vi "art联动采集V4.8.2.vi"() -> ()   [LabVIEW 2016]
uses:
  <vilib>/Instr/_visa.llb/VISA Configure Serial Port (Instr).vi
  <vilib>/Utility/file.llb/Write Delimited Spreadsheet (DBL).vi
panel:
  out "水平进度条":u8(slide) scale=0.0..100.0
  out "x+y 3":dbl=3.0
  in  "分层图查看":bool
  in  "hDevice 2":i32
  in  "逐行扫描":bool
  in  "定位模式":bool
  in  "X终点":dbl
  in  "Y终点":dbl
  in  "高级设置":bool
  in  "Y轴回零速度":dbl=15000.0
  in  "X轴回零速度":dbl=15000.0
  in  "细分设置":dbl=8.0
  in  "等待时间":u32=40
  in  "文件保存":path=path "C:/Users/H301/Desktop/art采集实验数据" caption="保存路径"
  out "已用时（s）":dbl format="%<%H:%M:%S>t"
  out "error out":errorcluster caption="错误输出"
  in  "退出扫描(Esc)":bool
  in  "N_Length":i32=16384
  out "M_Length":i32
  out "hDevice":i32=241832032
  out "pulDDR2Length":u32=256
  out "毫秒计时值":u32=3586537
  out "数组":dbl[][](array[numeric])=[[58819.77200735986, 88200.32943600747]]
  out "强度图":dbl[][](graph)=[[58819.77200735986, 88200.32943600747]]
  out "judge":dbl
  out "Xloop":dbl
  out "幅频谱":dbl[](graph)
  out "时域谱":dbl[](graph)
  out "错误输出":errorcluster
  in  "启动":bool
  in  "逐点扫描":bool
  in  "X归零":bool
  in  "Y归零":bool
  in  "Y起点":dbl
  in  "Y轴速度":dbl=9000.0
  in  "X轴速度":dbl=9000.0
  out "电机状态":bool
  in  "电机端口":refnum<visa-resource-name>="COM6"
  out "Yloop":dbl=1.0
  out "X扫描范围":dbl=150.0
  out "Y扫描范围":dbl=75.0
  out "Y序":i32
  in  "X起点":dbl
  out "Y(mm)":dbl
  out "x+y 2":dbl=3.0
  in  "Y:":dbl=1.0
  in  "精度":dbl=0.001
  in  "电机急停":bool
  out "X（mm）":dbl
  out "x+y":dbl=1.0
  in  "X:":dbl=1.0
  # "实时坐标"
  # "时域谱"
  # "频域谱"
  # "归零"
  # "扫描区域"
  # "扫描步进(mm)"
  # "X:"
  # "~"
  # "Y:"
  # "~"
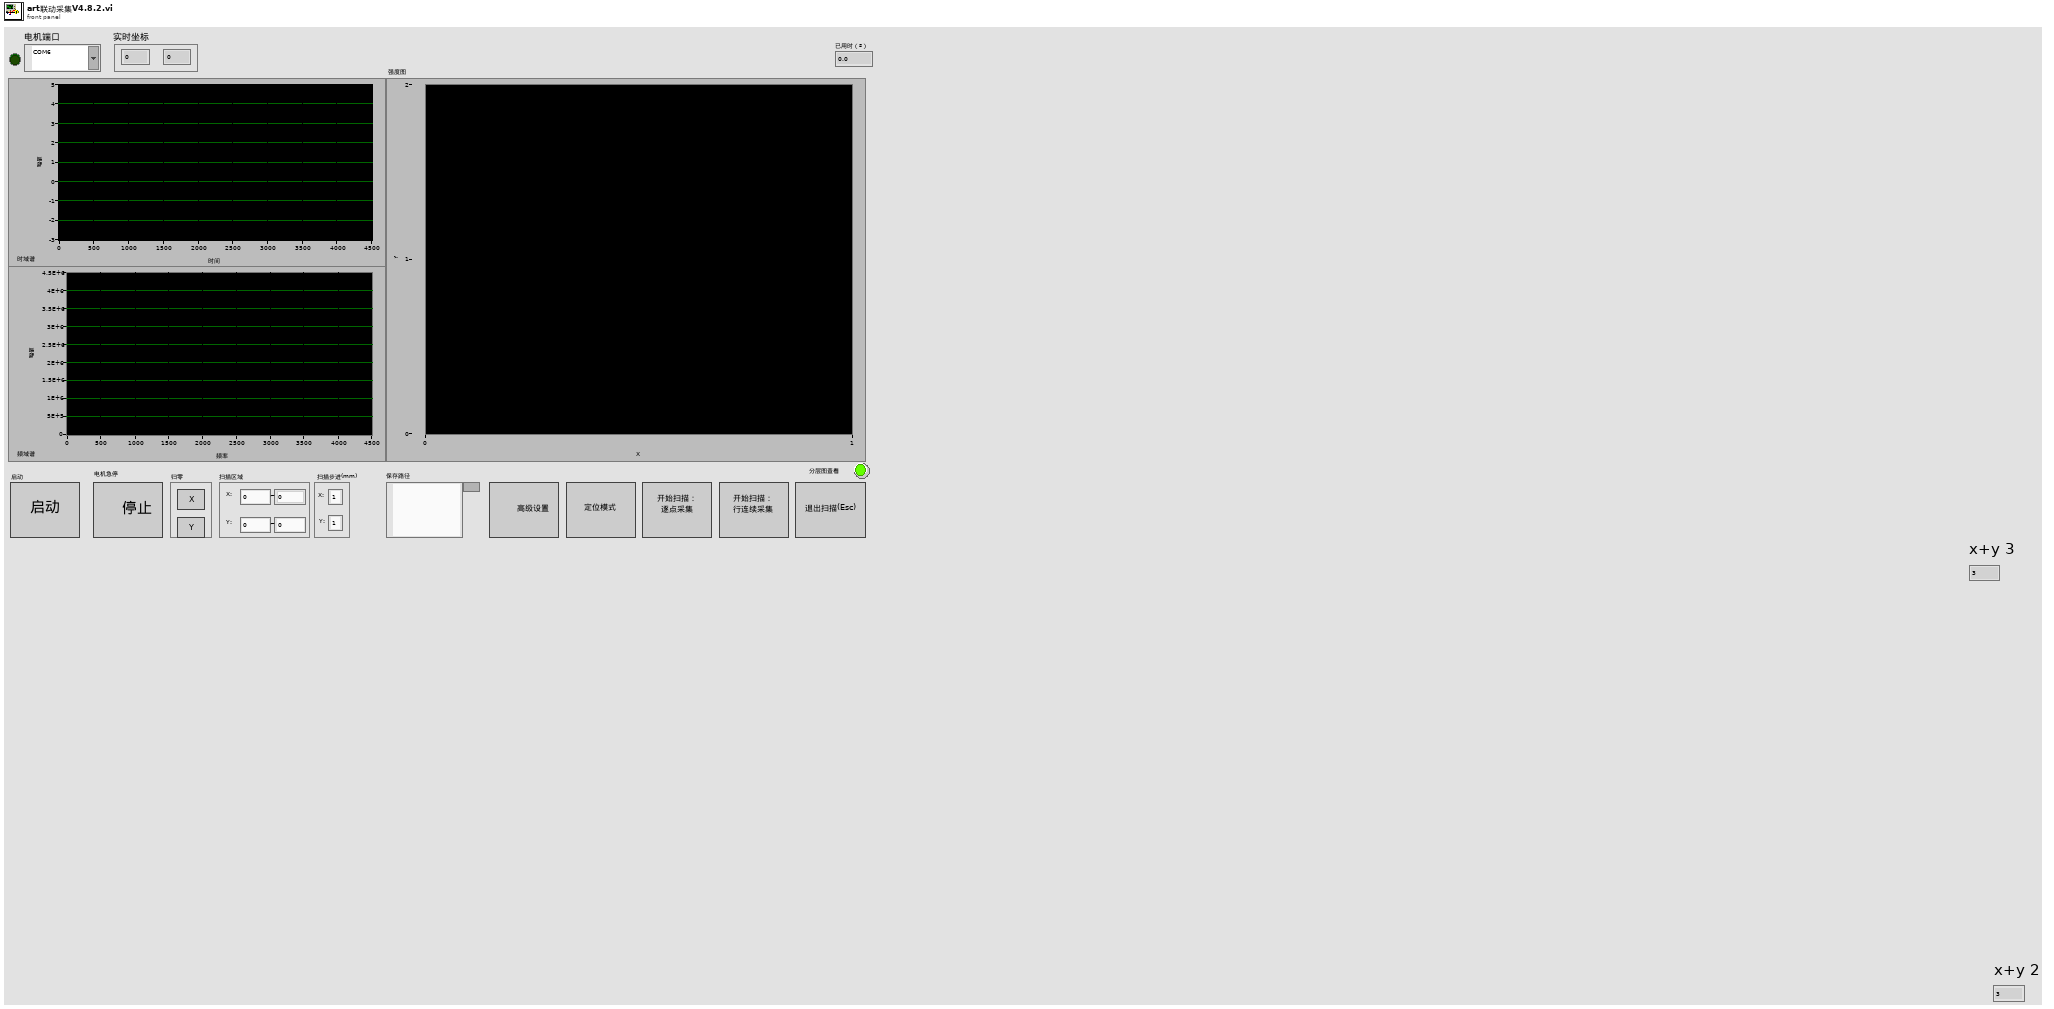
[diagram p1: front panel]
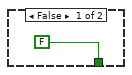
[diagram p2: hidden frame]
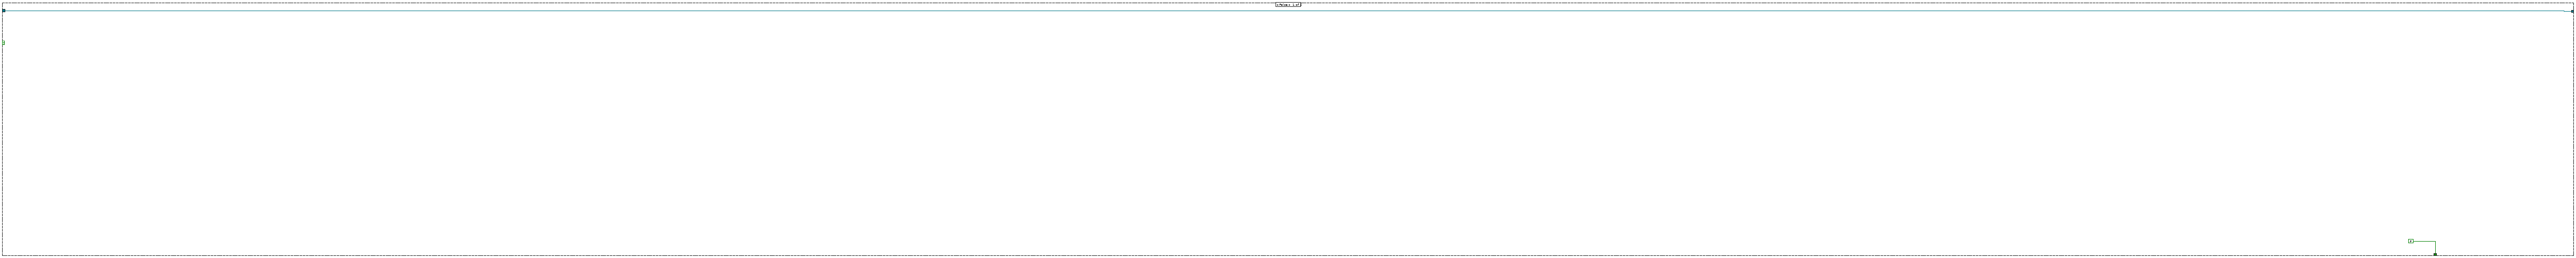
[diagram p3: hidden frame]
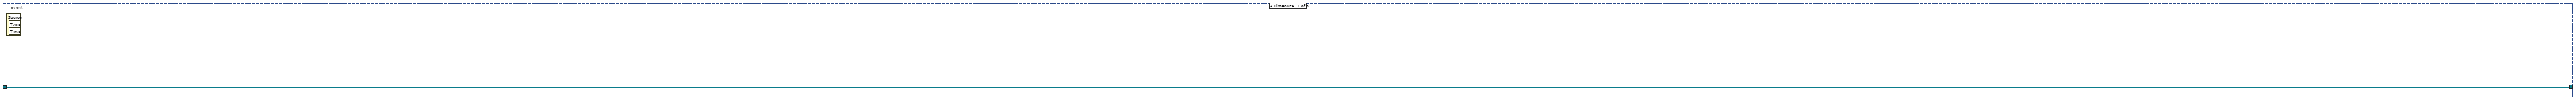
[diagram p4: hidden frame]
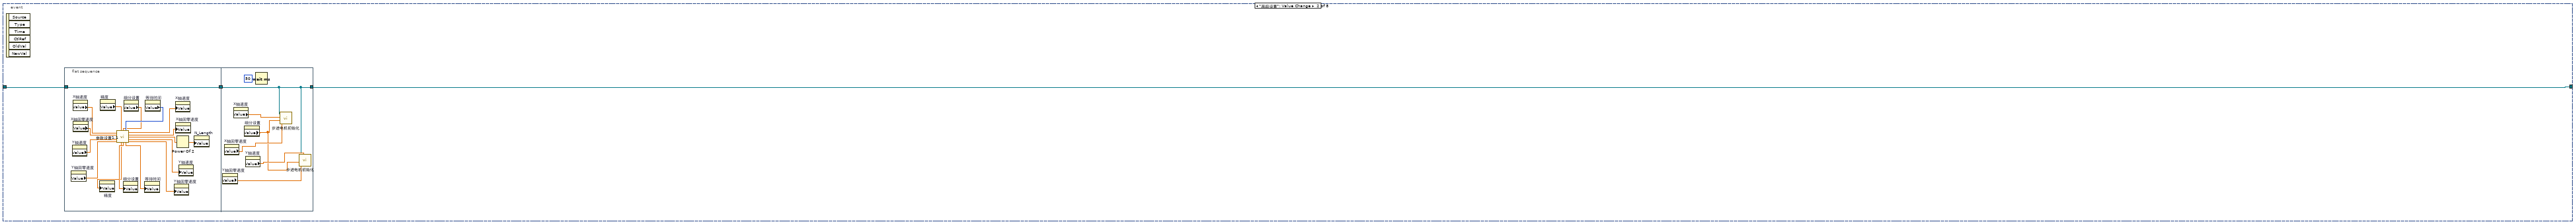
[diagram p5: hidden frame]
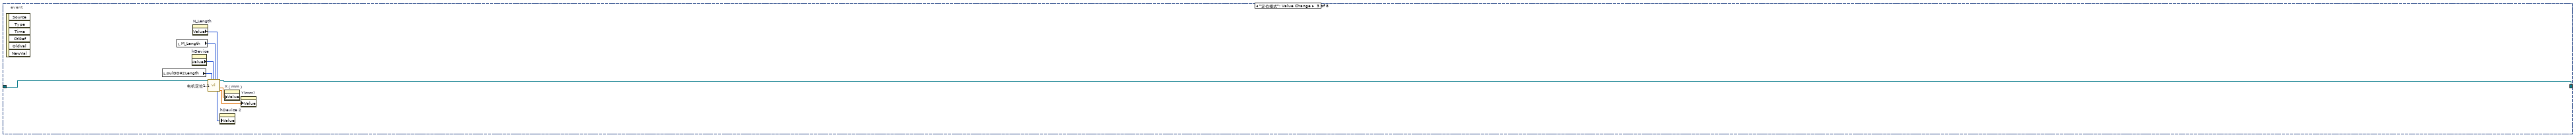
[diagram p6: hidden frame]
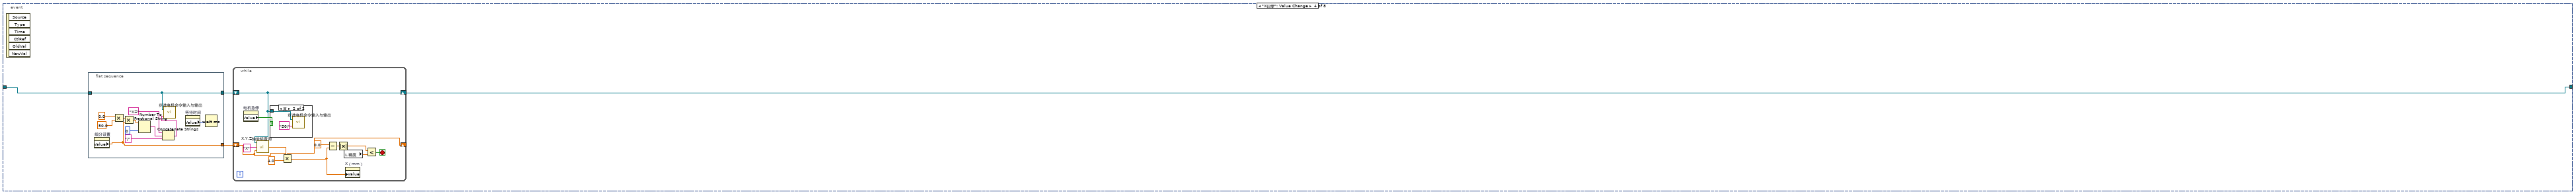
[diagram p7: hidden frame]
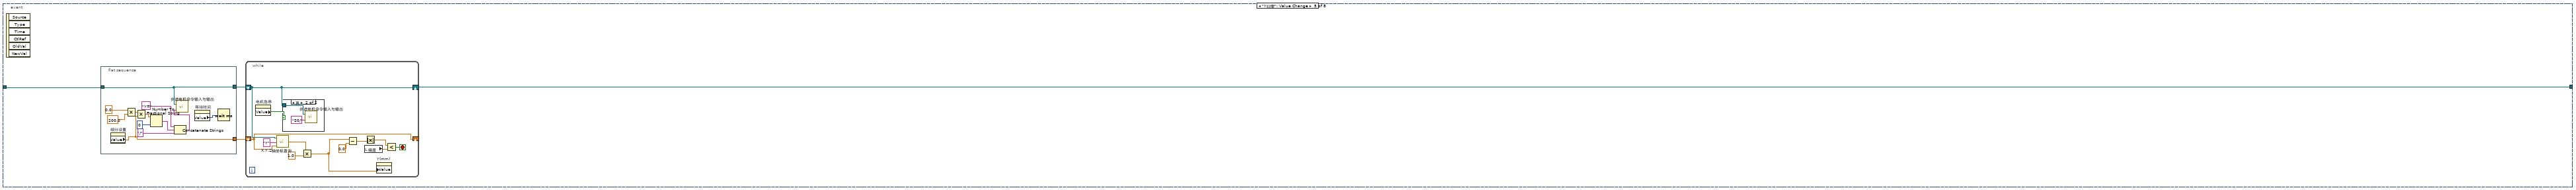
[diagram p9: hidden frame]
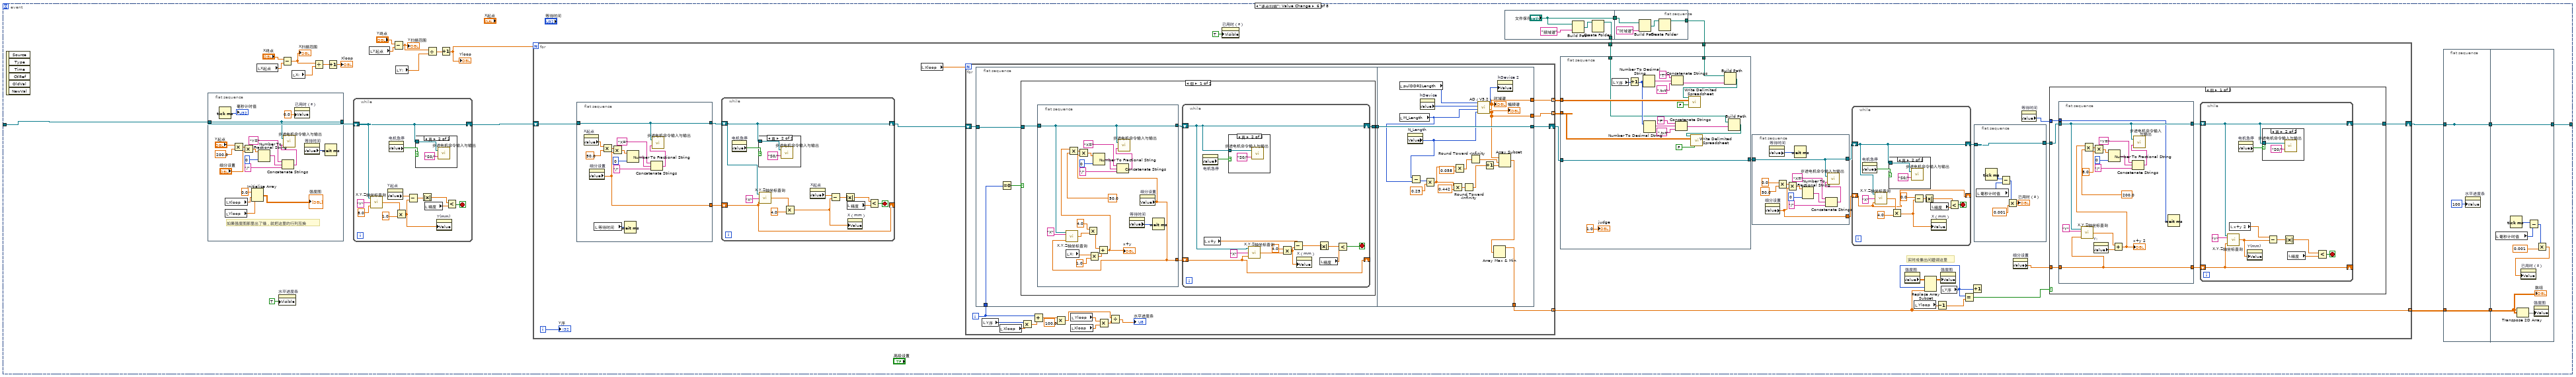
[diagram p11: hidden frame]
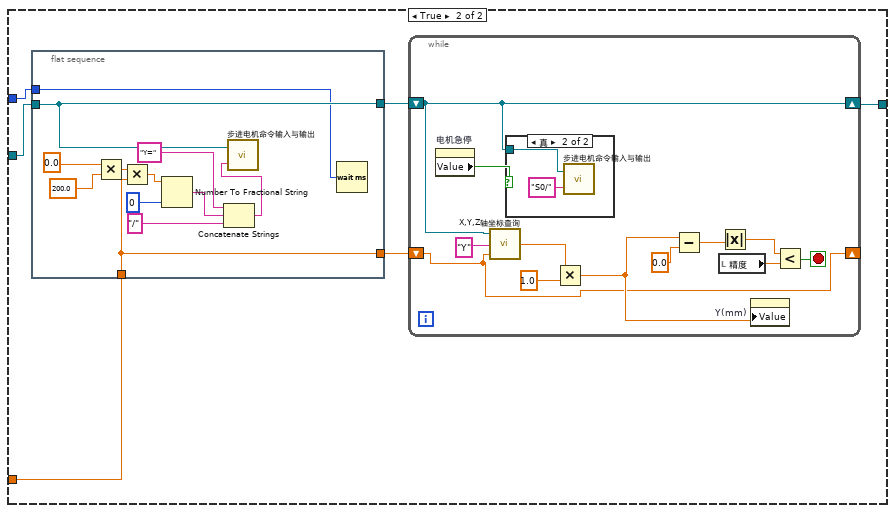
[diagram p16: hidden frame]
diagram:
  n1 = for {
    N: 255 -> [_]
    tunnel: [w12] -> w9 mode=indexing
    i -> [w12]
  }
  n2 = To Unsigned Byte Integer(number=w9) -> (unsigned 8bit integer=w6:u8[])
  n3 = Join Numbers(hi=u16 0, lo=w6) -> ((hi.lo)=w8:u32[])
  n4 = Join Numbers(hi=w6, lo=w6) -> ((hi.lo)=w5:u16[])
  n5 = Join Numbers(hi=w8, lo=w5) -> ((hi.lo)=w4:u64[])
  n6 = property on="强度图" class="IntGraph (严格)"("Color Table"=w4) -> ()  [unwired: 2 in, 2 out]
  n7 = property on="水平进度条" class="Slide (严格)"("Visible"=FALSE ("可见")) -> ()  [unwired: 2 in, 2 out]
  n8 = while {
    stop <- w13 stop-if-true
    n9 = case shown="真" "启动" {
      tunnel: [FALSE ("ESC") w21] -> w13
      frame False {
      }
      frame True {
        w32 = 0  # OutClockSource
        w33 = 0  # bClockSourceDir
        w35 = 10000000  # Frequency
        w36 = 0  # ClockSource
        w37 = 0  # TrigLevelVolt
        w25 = 1
        w38 = 0  # TriggerDir
        w39 = 0  # TriggerSource
        w40 = 0  # ATRTriggerChannel
        w41 = 0  # TriggerMode
        w26 = 0  # M_Length
        w42 = 1  # CouplingType
        w43 = 0  # DeviceLgcID
        w53 = u16 0 items=["无", "XON/XOFF", "RTS/CTS", "XON/XOFF & RTS/CTS", "DTR/DSR", "XON/XOFF & DTR/DSR"] ("flow control (0:none)")
        w54 = u16 10 items=["1.0"=10, "1.5"=15, "2.0"=20] ("stop bits (10: 1 bit)")
        # "3"
        # "2"
        # "1"
        n10 = call-poly "VISA Configure Serial Port"("VISA resource name"="电机端口", "baud rate (9600)"=u32 9600, "data bits (8)"=u16 8, "parity (0:none)"=enum16{"None", "Odd", "Even", "Mark", "Space"}."None", "stop bits (10: 1 bit)"=w54, "flow control (0:none)"=w53) -> ("VISA resource name out"=w45:refnum<visa-resource-name>, "error out"=→"error out":errorcluster)  [unwired: 1 in, 7 out]
        n11 = Build Array "InputRange"(w25, w25, w25, w25) -> (w24:i32[])
        n12 = dll-call lib="PTH2aabs CUsersH301Desktopart闭环扫描程序采集卡控制INFamd64PCI8502_32.dll" fn="PCI8502_CreateDevice" label="CreateDevice"("DeviceLgcID"=w43) -> (w30:i32)  [unwired: 4 in, 2 out]
        n13 = property on="细分设置" class="DigNum (严格)"() -> ("Value"=w20:dbl)  [unwired: 2 in, 2 out]
        n14 = Build Array (concatenate) "InitDeviceAD"(w35, w24, w42, w26, "N_Length", w41, w40, w39, w38, w37, w36, w33, w32) -> (w34:i32[])
        n15 = call "步进电机初始化.vi"("回零速度"="X轴回零速度", "细分设置"=w20, "X轴速度"="X轴速度", "串口通信端口"=w45) -> ()  [unwired: 2 in, 1 out]
        n16 = dll-call lib="PTH2aabs CUsersH301Desktopart闭环扫描程序采集卡控制INFamd64PCI8502_32.dll" fn="PCI8502_GetDDR2Length" label="GetDDR2Length"("hDevice"=w30, "pulDDR2Length"=u32 0) -> ("hDevice"=w29:i32, "pulDDR2Length"=→"pulDDR2Length":u32)  [unwired: 4 in, 2 out]
        n17 = call "步进电机初始化.vi"("Y轴速度"="Y轴速度", "回零速度"="Y轴回零速度", "细分设置"=w20, "串口通信端口"=w45) -> ()  [unwired: 2 in, 1 out]
        n18 = call "步进电机命令输入与输出.vi"("输入字符串"="?R/", "串口通信端口"=w45) -> ("返回字符串"=w50:string)
        n19 = dll-call lib="PTH2aabs CUsersH301Desktopart闭环扫描程序采集卡控制INFamd64PCI8502_32.dll" fn="PCI8502_InitDeviceAD" label="InitDeviceAD"("hDevice"=w29, "pADPara"=w34) -> ("hDevice"=→"hDevice":i32)  [unwired: 5 in, 2 out]
        n20 = String Subset(string=w50, offset (0)=0 ("偏移量(0)"), length (rest)=2 ("长度（剩余）")) -> (substring=w47:string)
        n21 = Equal?(x=w47, y="OK") -> (x = y?=w44:bool)
        "电机状态" <- w44
        n22 = case shown="真" w44 {
          tunnel: w45 -> [w65 w68]
          tunnel: [w65 w66] -> w22
          tunnel: [FALSE ("ESC") w67] -> w21
          frame False {
          }
          frame True {
            n23 = while {
              tunnel: ["退出扫描(Esc)"] -> w67
              shift-right: [w71] -> w66
              shift-left: w68 -> [w76]
              stop <- "退出扫描(Esc)" stop-if-true
              n24 = property on="水平进度条" class="Slide (严格)"("Visible"=FALSE ("可见")) -> ()  [unwired: 2 in, 2 out]
              n25 = property on="高级设置" class="Bool"("Visible"=TRUE ("可见")) -> ()  [unwired: 2 in, 2 out]
              n26 = property on="定位模式" class="Bool"("Visible"=TRUE ("可见")) -> ()  [unwired: 2 in, 2 out]
              n27 = property on="水平进度条" class="Slide (严格)"("Value"=u8 0 ("水平进度条")) -> ()  [unwired: 2 in, 2 out]
              n28 = event shown="[6] \"逐行扫描\": 值改变" {
                selector: _ -> [_ _ _ _ _ _ _ _]
                dyn-events: _ -> [_ _ _ _ _ _ _ _]
                timeout: 1 -> [_ _ _ _ _ _ _ _]
                tunnel: w76 -> [w77 w80 w113 w117 w147 w198 w507 w735]
                tunnel: [w77 w79 w112 w115 w145 w193 w510 w734] -> w71
                event Timeout {
                  n29 = event-data() -> ()  [unwired: 1 in, 3 out]
                }
                event "高级设置": Value Change {
                  n30 = event-data() -> ()  [unwired: 1 in, 6 out]
                  n31 = flat-sequence {
                    tunnel: w80 -> [w83]
                    tunnel: [w83] -> w78
                    tunnel: [w99] -> w79
                    tunnel: w78 -> [w99]
                    frame #0 {
                      n32 = property on="Y轴回零速度" class="DigNum (严格)"() -> ("Value"=w87:dbl)  [unwired: 2 in, 2 out]
                      n33 = property on="Y轴速度" class="DigNum (严格)"() -> ("Value"=w86:dbl)  [unwired: 2 in, 2 out]
                      n34 = property on="X轴速度" class="DigNum (严格)"() -> ("Value"=w84:dbl)  [unwired: 2 in, 2 out]
                      n35 = property on="X轴回零速度" class="DigNum (严格)"() -> ("Value"=w85:dbl)  [unwired: 2 in, 2 out]
                      n36 = property on="精度" class="DigNum (严格)"() -> ("Value"=w91:dbl)  [unwired: 2 in, 2 out]
                      n37 = property on="细分设置" class="DigNum (严格)"() -> ("Value"=w92:dbl)  [unwired: 2 in, 2 out]
                      n38 = property on="等待时间" class="DigNum (严格)"() -> ("Value"=w93:u32)  [unwired: 2 in, 2 out]
                      n39 = call "参数设置1.1.vi"("X轴速度"=w84, "精度"=w91, "细分设置"=w92, "等待时间"=w93, "X轴回零速度"=w85, "Y轴速度"=w86, "Y轴回零速度"=w87) -> ("X轴速度"=w94:dbl, "X轴回零速度"=w95:dbl, "采样阶"=w81:dbl, "Y轴速度"=w96:dbl, "精度"=w88:dbl, "细分设置"=w89:dbl, "等待时间"=w90:dbl, "Y轴回零速度"=w97:dbl)  [unwired: 1 in]
                      n40 = property on="精度" class="DigNum (严格)"("Value"=w88) -> ()  [unwired: 2 in, 2 out]
                      n41 = property on="细分设置" class="DigNum (严格)"("Value"=w89) -> ()  [unwired: 2 in, 2 out]
                      n42 = property on="等待时间" class="DigNum (严格)"("Value"=w90) -> ()  [unwired: 2 in, 2 out]
                      n43 = property on="Y轴回零速度" class="DigNum (严格)"("Value"=w97) -> ()  [unwired: 2 in, 2 out]
                      n44 = property on="X轴速度" class="DigNum (严格)"("Value"=w94) -> ()  [unwired: 2 in, 2 out]
                      n45 = property on="X轴回零速度" class="DigNum (严格)"("Value"=w95) -> ()  [unwired: 2 in, 2 out]
                      n46 = Power Of 2(x=w81) -> (2^x=w82:dbl)
                      n47 = property on="Y轴速度" class="DigNum (严格)"("Value"=w96) -> ()  [unwired: 2 in, 2 out]
                      n48 = property on="N_Length" class="DigNum (严格)"("Value"=w82) -> ()  [unwired: 2 in, 2 out]
                    }
                    frame #1 {
                      n49 = property on="Y轴回零速度" class="DigNum (严格)"() -> ("Value"=w103:dbl)  [unwired: 2 in, 2 out]
                      n50 = property on="X轴回零速度" class="DigNum (严格)"() -> ("Value"=w102:dbl)  [unwired: 2 in, 2 out]
                      n51 = property on="X轴速度" class="DigNum (严格)"() -> ("Value"=w101:dbl)  [unwired: 2 in, 2 out]
                      n52 = property on="细分设置" class="DigNum (严格)"() -> ("Value"=w100:dbl)  [unwired: 2 in, 2 out]
                      n53 = property on="Y轴速度" class="DigNum (严格)"() -> ("Value"=w104:dbl)  [unwired: 2 in, 2 out]
                      n54 = Wait (ms)(milliseconds to wait=u32 50 ("等待时间（毫秒）")) -> ()  [unwired: 1 out]
                      n55 = call "步进电机初始化.vi"("回零速度"=w102, "细分设置"=w100, "X轴速度"=w101, "串口通信端口"=w99) -> ()  [unwired: 2 in, 1 out]
                      n56 = call "步进电机初始化.vi"("Y轴速度"=w104, "回零速度"=w103, "细分设置"=w100, "串口通信端口"=w99) -> ()  [unwired: 2 in, 1 out]
                    }
                  }
                }
                event "定位模式": Value Change {
                  n57 = event-data() -> ()  [unwired: 1 in, 6 out]
                  n58 = local read "pulDDR2Length"() -> (w109:u32)
                  n59 = local read "M_Length"() -> (w107:i32)
                  n60 = property on="hDevice" class="DigNum (严格)"() -> ("Value"=w108:i32)  [unwired: 2 in, 2 out]
                  n61 = property on="N_Length" class="DigNum (严格)"() -> ("Value"=w106:i32)  [unwired: 2 in, 2 out]
                  n62 = call "电机定位1.1.vi"("VISA I"=w113, "pulDDR2Length"=w109, "hDevice"=w108, "M-length"=w107, "N-length"=w106) -> ("hDevice out"=w105:i32, "VISA O"=w112:refnum<visa-resource-name>, "X"=w111:dbl, "Y"=w110:dbl)  [unwired: 11 in]
                  n63 = property on="hDevice 2" class="DigNum (严格)"("Value"=w105) -> ()  [unwired: 2 in, 2 out]
                  n64 = property on="X（mm）" class="DigNum (严格)"("Value"=w111) -> ()  [unwired: 2 in, 2 out]
                  n65 = property on="Y(mm)" class="DigNum (严格)"("Value"=w110) -> ()  [unwired: 2 in, 2 out]
                }
                event "X归零": Value Change {
                  n66 = event-data() -> ()  [unwired: 1 in, 6 out]
                  n67 = flat-sequence {
                    tunnel: w117 -> [w121]
                    tunnel: [w121] -> w116
                    tunnel: [w118] -> w114
                    frame #0 {
                      n68 = property on="细分设置" class="DigNum (严格)"() -> ("Value"=w118:dbl)  [unwired: 2 in, 2 out]
                      n69 = Multiply(x=0.0, y=50.0) -> (x*y=w124:dbl)
                      n70 = Multiply(x=w124, y=w118) -> (x*y=w129:dbl)
                      n71 = Number To Fractional String(number=w129, precision (6)=i16 0 ("精度(6)")) -> (F-format string=w127:string)  [unwired: 2 out]
                      n72 = Concatenate Strings("X=" ("字符串"), w127, "/" ("字符串")) -> (w122:string)
                      n73 = call "步进电机命令输入与输出.vi"("输入字符串"=w122, "串口通信端口"=w121) -> ()  [unwired: 1 out]
                      n74 = property on="等待时间" class="DigNum (严格)"() -> ("Value"=w119:u32)  [unwired: 2 in, 2 out]
                      n75 = Wait (ms)(milliseconds to wait=w119) -> ()  [unwired: 1 out]
                    }
                  }
                  n76 = while {
                    shift-right: [w131] -> w115
                    shift-left: w116 -> [w131]
                    shift-right: [w130] -> _
                    shift-left: w114 -> [w130]
                    stop <- w137 stop-if-true
                    n77 = property on="电机急停" class="Bool (严格)"() -> ("Value"=w138:bool)  [unwired: 2 in, 2 out]
                    n78 = call "X,Y,Z轴坐标查询.vi"("细分设置"=w130, "查询坐标轴"="X", "串口通信端口"=w131) -> ("坐标(mm)"=w139:dbl)
                    n79 = case shown="真" w138 {
                      tunnel: w131 -> [_ w142]
                      frame False {
                      }
                      frame True {
                        n80 = call "步进电机命令输入与输出.vi"("输入字符串"="S0/", "串口通信端口"=w142) -> ()  [unwired: 1 out]
                      }
                    }
                    n81 = Multiply(x=w139, y=4.0 ("x")) -> (x*y=w135:dbl)
                    n82 = Subtract(x=0.0, y=w135) -> (x-y=w134:dbl)
                    n83 = Absolute Value(x=w134) -> (abs(x)=w133:dbl)
                    n84 = local read "精度"() -> (w136:dbl)
                    n85 = property on="X（mm）" class="DigNum (严格)"("Value"=w135) -> ()  [unwired: 2 in, 2 out]
                    n86 = Less?(x=w133, y=w136) -> (x < y?=w137:bool)
                  }
                }
                event "Y归零": Value Change {
                  n87 = event-data() -> ()  [unwired: 1 in, 6 out]
                  n88 = flat-sequence {
                    tunnel: w147 -> [w151]
                    tunnel: [w151] -> w146
                    tunnel: [w148] -> w144
                    frame #0 {
                      n89 = property on="细分设置" class="DigNum (严格)"() -> ("Value"=w148:dbl)  [unwired: 2 in, 2 out]
                      n90 = Multiply(x=0.0, y=200.0) -> (x*y=w154:dbl)
                      n91 = Multiply(x=w154, y=w148) -> (x*y=w159:dbl)
                      n92 = Number To Fractional String(number=w159, precision (6)=i16 0 ("精度(6)")) -> (F-format string=w157:string)  [unwired: 2 out]
                      n93 = Concatenate Strings("Y=" ("字符串"), w157, "/" ("字符串")) -> (w152:string)
                      n94 = call "步进电机命令输入与输出.vi"("输入字符串"=w152, "串口通信端口"=w151) -> ()  [unwired: 1 out]
                      n95 = property on="等待时间" class="DigNum (严格)"() -> ("Value"=w149:u32)  [unwired: 2 in, 2 out]
                      n96 = Wait (ms)(milliseconds to wait=w149) -> ()  [unwired: 1 out]
                    }
                  }
                  n97 = while {
                    shift-right: [w161] -> w145
                    shift-left: w146 -> [w161]
                    shift-right: [w160] -> _
                    shift-left: w144 -> [w160]
                    stop <- w167 stop-if-true
                    n98 = property on="电机急停" class="Bool (严格)"() -> ("Value"=w168:bool)  [unwired: 2 in, 2 out]
                    n99 = call "X,Y,Z轴坐标查询.vi"("细分设置"=w160, "查询坐标轴"="Y", "串口通信端口"=w161) -> ("坐标(mm)"=w169:dbl)
                    n100 = case shown="真" w168 {
                      tunnel: w161 -> [_ w172]
                      frame False {
                      }
                      frame True {
                        n101 = call "步进电机命令输入与输出.vi"("输入字符串"="S0/", "串口通信端口"=w172) -> ()  [unwired: 1 out]
                      }
                    }
                    n102 = Multiply(x=w169, y=1.0 ("x")) -> (x*y=w165:dbl)
                    n103 = Subtract(x=w165, y=0.0 ("x")) -> (x-y=w163:dbl)
                    n104 = local read "精度"() -> (w166:dbl)
                    n105 = Absolute Value(x=w163) -> (abs(x)=w162:dbl)
                    n106 = property on="Y(mm)" class="DigNum (严格)"("Value"=w165) -> ()  [unwired: 2 in, 2 out]
                    n107 = Less?(x=w162, y=w166) -> (x < y?=w167:bool)
                  }
                }
                event "逐点扫描": Value Change {
                  n108 = event-data() -> ()  [unwired: 1 in, 6 out]
                  n109 = flat-sequence {
                    tunnel: w198 -> [w227]
                    tunnel: [w227] -> w189
                    frame #0 {
                      # "如果强度图那里出了错，就把这里的行列互换"
                      n110 = Tick Count (ms)() -> (millisecond timer value=→"毫秒计时值":u32)
                      n111 = local read "Xloop"() -> (w222:dbl)
                      n112 = local read "Yloop"() -> (w221:dbl)
                      n113 = Multiply(x="Y起点", y=200.0) -> (x*y=w230:dbl)
                      n114 = Multiply(x=w230, y="细分设置") -> (x*y=w235:dbl)
                      n115 = Initialize Array(0.0 ("元素"), w222, w221) -> (→"强度图":dbl[][])
                      n116 = Number To Fractional String(number=w235, precision (6)=i16 0 ("精度(6)")) -> (F-format string=w233:string)  [unwired: 2 out]
                      n117 = Concatenate Strings("Y=" ("字符串"), w233, "/" ("字符串")) -> (w228:string)
                      n118 = call "步进电机命令输入与输出.vi"("输入字符串"=w228, "串口通信端口"=w227) -> ()  [unwired: 1 out]
                      n119 = property on="已用时（s）" class="DigNum (严格)"("Value"=0.0 ("已用时（s）")) -> ()  [unwired: 2 in, 2 out]
                      n120 = property on="等待时间" class="DigNum (严格)"() -> ("Value"=w219:u32)  [unwired: 2 in, 2 out]
                      n121 = Wait (ms)(milliseconds to wait=w219) -> ()  [unwired: 1 out]
                    }
                  }
                  n122 = local read "X起点"() -> (w185:dbl)
                  n123 = property on="水平进度条" class="Slide (严格)"("Visible"=TRUE ("可见")) -> ()  [unwired: 2 in, 2 out]
                  n124 = Subtract(x="X终点", y=w185) -> (x-y=w184:dbl)
                  "X扫描范围" <- w184
                  n125 = local read "X:"() -> (w192:dbl)
                  n126 = Divide(x=w184, y=w192) -> (x/y=w190:dbl)
                  n127 = Increment(x=w190) -> (x+1=→"Xloop":dbl)
                  n128 = while {
                    shift-right: [w236] -> w181
                    shift-left: w189 -> [w236]
                    stop <- w241 stop-if-true
                    n129 = call "X,Y,Z轴坐标查询.vi"("细分设置"=8.0, "查询坐标轴"="Y", "串口通信端口"=w236) -> ("坐标(mm)"=w243:dbl)
                    n130 = property on="Y起点" class="DigNum (严格)"() -> ("Value"=w245:dbl)  [unwired: 2 in, 2 out]
                    n131 = property on="电机急停" class="Bool (严格)"() -> ("Value"=w242:bool)  [unwired: 2 in, 2 out]
                    n132 = Multiply(x=w243, y=1.0 ("x")) -> (x*y=w239:dbl)
                    n133 = Subtract(x=w245, y=w239) -> (x-y=w238:dbl)
                    n134 = case shown="真" w242 {
                      tunnel: w236 -> [_ w248]
                      frame False {
                      }
                      frame True {
                        n135 = call "步进电机命令输入与输出.vi"("输入字符串"="S0/", "串口通信端口"=w248) -> ()  [unwired: 1 out]
                      }
                    }
                    n136 = Absolute Value(x=w238) -> (abs(x)=w237:dbl)
                    n137 = local read "精度"() -> (w240:dbl)
                    n138 = property on="Y(mm)" class="DigNum (严格)"("Value"=w239) -> ()  [unwired: 2 in, 2 out]
                    n139 = Less?(x=w237, y=w240) -> (x < y?=w241:bool)
                  }
                  n140 = local read "Y起点"() -> (w187:dbl)
                  n141 = Subtract(x="Y终点", y=w187) -> (x-y=w183:dbl)
                  "Y扫描范围" <- w183
                  n142 = local read "Y:"() -> (w197:dbl)
                  n143 = Divide(x=w183, y=w197) -> (x/y=w196:dbl)
                  n144 = Increment(x=w196) -> (x+1=w195:dbl)
                  "Yloop" <- w195
                  n145 = for {
                    N: w195 -> [_]
                    shift-right: [w273] -> w174
                    shift-left: w181 -> [w254]
                    tunnel: [w256] -> w194 mode=indexing
                    tunnel: w179 -> [w260]
                    tunnel: w182 -> [w259]
                    i -> [w274]
                    # "实时成像出问题调这里"
                    n146 = flat-sequence {
                      tunnel: w254 -> [w331]
                      tunnel: [w331] -> w272
                      tunnel: [w330] -> w264
                      frame #0 {
                        n147 = property on="X起点" class="DigNum (严格)"() -> ("Value"=w328:dbl)  [unwired: 2 in, 2 out]
                        n148 = property on="细分设置" class="DigNum (严格)"() -> ("Value"=w330:dbl)  [unwired: 2 in, 2 out]
                        n149 = local read "等待时间"() -> (w329:u32)
                        n150 = Multiply(x=w328, y=50.0) -> (x*y=w334:dbl)
                        n151 = Multiply(x=w334, y=w330) -> (x*y=w339:dbl)
                        n152 = Wait (ms)(milliseconds to wait=w329) -> ()  [unwired: 1 out]
                        n153 = Number To Fractional String(number=w339, precision (6)=i16 0 ("精度(6)")) -> (F-format string=w337:string)  [unwired: 2 out]
                        n154 = Concatenate Strings("X=" ("字符串"), w337, "/" ("字符串")) -> (w332:string)
                        n155 = call "步进电机命令输入与输出.vi"("输入字符串"=w332, "串口通信端口"=w331) -> ()  [unwired: 1 out]
                      }
                    }
                    n156 = while {
                      shift-right: [w341] -> w252
                      shift-left: w272 -> [w341]
                      shift-right: [w340] -> _
                      shift-left: w264 -> [w340]
                      stop <- w346 stop-if-true
                      n157 = property on="电机急停" class="Bool (严格)"() -> ("Value"=w347:bool)  [unwired: 2 in, 2 out]
                      n158 = case shown="真" w347 {
                        tunnel: w341 -> [_ w352]
                        frame False {
                        }
                        frame True {
                          n159 = call "步进电机命令输入与输出.vi"("输入字符串"="S0/", "串口通信端口"=w352) -> ()  [unwired: 1 out]
                        }
                      }
                      n160 = call "X,Y,Z轴坐标查询.vi"("细分设置"=w340, "查询坐标轴"="X", "串口通信端口"=w341) -> ("坐标(mm)"=w348:dbl)
                      n161 = Multiply(x=w348, y=4.0 ("x")) -> (x*y=w344:dbl)
                      n162 = property on="X起点" class="DigNum (严格)"() -> ("Value"=w350:dbl)  [unwired: 2 in, 2 out]
                      n163 = Subtract(x=w350, y=w344) -> (x-y=w343:dbl)
                      n164 = Absolute Value(x=w343) -> (abs(x)=w342:dbl)
                      n165 = local read "精度"() -> (w345:dbl)
                      n166 = property on="X（mm）" class="DigNum (严格)"("Value"=w344) -> ()  [unwired: 2 in, 2 out]
                      n167 = Less?(x=w342, y=w345) -> (x < y?=w346:bool)
                    }
                    n168 = local read "Xloop"() -> (w265:dbl)
                    n169 = for {
                      N: w265 -> [_]
                      shift-right: [w435] -> w253
                      shift-left: w252 -> [w431]
                      tunnel: [w434] -> w271 mode=indexing
                      tunnel: [w433] -> w270 mode=indexing
                      tunnel: [w432] -> w256 mode=indexing
                      i -> [w423]
                      n170 = flat-sequence {
                        tunnel: w431 -> [w440]
                        tunnel: [w439] -> w436
                        tunnel: w423 -> [w437]
                        tunnel: [w498] -> w435
                        tunnel: w436 -> [w498]
                        tunnel: [w497] -> w434
                        tunnel: [w496] -> w433
                        tunnel: [w494] -> w432
                        frame #0 {
                          n171 = Equal To 0?(x=w437) -> (x = 0?=w438:bool)
                          n172 = case shown="假" w438 {
                            tunnel: w440 -> [w443 w478]
                            tunnel: [w442 w478] -> w439
                            frame False {
                              n173 = flat-sequence {
                                tunnel: w443 -> [w453]
                                tunnel: [w453] -> w444
                                tunnel: [w445] -> w441
                                frame #0 {
                                n174 = local read "X:"() -> (w447:dbl)
                                n175 = Multiply(x=w447, y=1.0 ("x")) -> (x*y=w452:dbl)
                                n176 = property on="等待时间" class="DigNum (严格)"() -> ("Value"=w446:u32)  [unwired: 2 in, 2 out]
                                n177 = property on="细分设置" class="DigNum (严格)"() -> ("Value"=w445:dbl)  [unwired: 2 in, 2 out]
                                n178 = call "X,Y,Z轴坐标查询.vi"("细分设置"=w445, "查询坐标轴"="X", "串口通信端口"=w453) -> ("坐标(mm)"=w449:dbl)
                                n179 = Multiply(x=4.0, y=w449) -> (x*y=w448:dbl)
                                n180 = Add(x=w448, y=w452) -> (x+y=w455:dbl)
                                "x+y" <- w455
                                n181 = Multiply(x=w455, y=50.0) -> (x*y=w458:dbl)
                                n182 = Multiply(x=w458, y=w445) -> (x*y=w463:dbl)
                                n183 = Number To Fractional String(number=w463, precision (6)=i16 0 ("精度(6)")) -> (F-format string=w461:string)  [unwired: 2 out]
                                n184 = Concatenate Strings("X=" ("字符串"), w461, "/" ("字符串")) -> (w456:string)
                                n185 = call "步进电机命令输入与输出.vi"("输入字符串"=w456, "串口通信端口"=w453) -> ()  [unwired: 1 out]
                                n186 = Wait (ms)(milliseconds to wait=w446) -> ()  [unwired: 1 out]
                                }
                              }
                              n187 = while {
                                shift-right: [w473] -> w442
                                shift-left: w444 -> [w473]
                                shift-right: [w464] -> _
                                shift-left: w441 -> [w464]
                                stop <- w472 stop-if-true
                                n188 = property on="电机急停" class="Bool (严格)"() -> ("Value"=w470:bool)  [unwired: 2 in, 2 out]
                                n189 = local read "x+y"() -> (w474:dbl)
                                n190 = case shown="真" w470 {
                                tunnel: w473 -> [_ w476]
                                frame False {
                                }
                                frame True {
                                n191 = call "步进电机命令输入与输出.vi"("输入字符串"="S0/", "串口通信端口"=w476) -> ()  [unwired: 1 out]
                                }
                                }
                                n192 = call "X,Y,Z轴坐标查询.vi"("细分设置"=w464, "查询坐标轴"="X", "串口通信端口"=w473) -> ("坐标(mm)"=w468:dbl)
                                n193 = Multiply(x=4.0, y=w468) -> (x*y=w467:dbl)
                                n194 = Subtract(x=w474, y=w467) -> (x-y=w466:dbl)
                                n195 = property on="X（mm）" class="DigNum (严格)"("Value"=w467) -> ()  [unwired: 2 in, 2 out]
                                n196 = Absolute Value(x=w466) -> (abs(x)=w465:dbl)
                                n197 = local read "精度"() -> (w469:dbl)
                                n198 = Less?(x=w465, y=w469) -> (x < y?=w472:bool)
                              }
                            }
                            frame True {
                            }
                          }
                        }
                        frame #1 {
                          n199 = local read "pulDDR2Length"() -> (w493:u32)
                          n200 = local read "M_Length"() -> (w492:i32)
                          n201 = property on="N_Length" class="DigNum (严格)"() -> ("Value"=w481:i32)  [unwired: 2 in, 2 out]
                          n202 = Subtract(x=w481, y=w492) -> (x-y=w490:i32)
                          n203 = property on="hDevice" class="DigNum (严格)"() -> ("Value"=w479:i32)  [unwired: 2 in, 2 out]
                          n204 = Multiply(x=w490, y=0.25) -> (x*y=w483:dbl)
                          n205 = Multiply(x=w483, y=0.442) -> (x*y=w485:dbl)
                          n206 = Multiply(x=w483, y=0.058) -> (x*y=w487:dbl)
                          n207 = Round Toward -Infinity(1:w485) -> (0:w482:dbl)
                          n208 = Round Toward -Infinity(1:w487) -> (0:w486:dbl)
                          n209 = call "AD（V3.2）.vi"("N-length"=w481, "M-length"=w492, "hDevice"=w479, "pulDDR2Length"=w493) -> ("幅频谱"=w496:dbl[], "时域谱"=w497:dbl[], "hDevice out"=w480:i32)  [unwired: 5 in]
                          "时域谱" <- w497
                          "幅频谱" <- w496
                          n210 = Increment(x=w482) -> (x+1=w489:dbl)
                          n211 = property on="hDevice 2" class="DigNum (严格)"("Value"=w480) -> ()  [unwired: 2 in, 2 out]
                          n212 = Array Subset(array=w496, index=w486, length=w489) -> (w495:dbl[])
                          n213 = Array Max & Min(array=w495) -> (max value=w494:dbl)  [unwired: 3 out]
                        }
                      }
                      n214 = local read "Y序"() -> (w425:i32)
                      n215 = local read "Xloop"() -> (w426:dbl)
                      n216 = Multiply(x=w425, y=w426) -> (x*y=w424:dbl)
                      n217 = Add(x=w423, y=w424) -> (x+y=w422:dbl)
                      n218 = Multiply(x=w422, y=100.0) -> (x*y=w420:dbl)
                      n219 = local read "Xloop"() -> (w430:dbl)
                      n220 = local read "Yloop"() -> (w429:dbl)
                      n221 = Multiply(x=w429, y=w430) -> (x*y=w428:dbl)
                      n222 = Divide(x=w420, y=w428) -> (x/y=→"水平进度条":dbl)
                    }
                    n223 = flat-sequence {
                      tunnel: w270 -> [w314]
                      tunnel: w271 -> [w322]
                      tunnel: w253 -> [w326]
                      tunnel: [w326] -> w266
                      tunnel: w260 -> [w309]
                      tunnel: w259 -> [w308]
                      frame #0 {
                        n224 = local read "Y序"() -> (w310:i32)
                        n225 = Increment(x=w310) -> (x+1=w311:i32)
                        n226 = Number To Decimal String(number=w311) -> (decimal integer string=w320:string)  [unwired: 1 in]
                        n227 = Number To Decimal String(number=w311) -> (decimal integer string=w319:string)  [unwired: 1 in]
                        n228 = Concatenate Strings("T" ("字符串"), w320, ".txt" ("字符串")) -> (w323:string)
                        n229 = Concatenate Strings("F" ("字符串"), w319, ".txt" ("字符串")) -> (w317:string)
                        n230 = Build Path(base path=w309, name or relative path=w323) -> (appended path=w325:path)
                        n231 = call-poly <vilib>:"Write Delimited Spreadsheet.vi"("file path (dialog if empty)"=w325, "2D data"=w322, "transpose? (no:F)"=FALSE) -> ()  [unwired: 11 in, 2 out]
                        n232 = Build Path(base path=w308, name or relative path=w317) -> (appended path=w315:path)
                        n233 = call-poly <vilib>:"Write Delimited Spreadsheet.vi"("file path (dialog if empty)"=w315, "2D data"=w314, "transpose? (no:F)"=FALSE) -> ()  [unwired: 11 in, 2 out]
                        "judge" <- 1.0
                      }
                    }
                    n234 = flat-sequence {
                      tunnel: w266 -> [w285]
                      tunnel: [w285] -> w267
                      tunnel: [w283] -> w263
                      frame #0 {
                        n235 = property on="细分设置" class="DigNum (严格)"() -> ("Value"=w283:dbl)  [unwired: 2 in, 2 out]
                        n236 = property on="等待时间" class="DigNum (严格)"() -> ("Value"=w282:u32)  [unwired: 2 in, 2 out]
                        n237 = Multiply(x=0.0, y=50.0) -> (x*y=w288:dbl)
                        n238 = Multiply(x=w288, y=w283) -> (x*y=w293:dbl)
                        n239 = Wait (ms)(milliseconds to wait=w282) -> ()  [unwired: 1 out]
                        n240 = Number To Fractional String(number=w293, precision (6)=i16 0 ("精度(6)")) -> (F-format string=w291:string)  [unwired: 2 out]
                        n241 = Concatenate Strings("X=" ("字符串"), w291, "/" ("字符串")) -> (w286:string)
                        n242 = call "步进电机命令输入与输出.vi"("输入字符串"=w286, "串口通信端口"=w285) -> ()  [unwired: 1 out]
                      }
                    }
                    n243 = while {
                      shift-right: [w295] -> w251
                      shift-left: w267 -> [w295]
                      shift-right: [w294] -> _
                      shift-left: w263 -> [w294]
                      stop <- w301 stop-if-true
                      n244 = property on="电机急停" class="Bool (严格)"() -> ("Value"=w302:bool)  [unwired: 2 in, 2 out]
                      n245 = call "X,Y,Z轴坐标查询.vi"("细分设置"=w294, "查询坐标轴"="X", "串口通信端口"=w295) -> ("坐标(mm)"=w303:dbl)
                      n246 = case shown="真" w302 {
                        tunnel: w295 -> [_ w306]
                        frame False {
                        }
                        frame True {
                          n247 = call "步进电机命令输入与输出.vi"("输入字符串"="S0/", "串口通信端口"=w306) -> ()  [unwired: 1 out]
                        }
                      }
                      n248 = Multiply(x=w303, y=4.0 ("x")) -> (x*y=w299:dbl)
                      n249 = Subtract(x=0.0, y=w299) -> (x-y=w298:dbl)
                      n250 = Absolute Value(x=w298) -> (abs(x)=w297:dbl)
                      n251 = local read "精度"() -> (w300:dbl)
                      n252 = property on="X（mm）" class="DigNum (严格)"("Value"=w299) -> ()  [unwired: 2 in, 2 out]
                      n253 = Less?(x=w297, y=w300) -> (x < y?=w301:bool)
                    }
                    n254 = property on="强度图" class="IntGraph (严格)"() -> ("Value"=w257:dbl[][])  [unwired: 2 in, 2 out]
                    n255 = local read "Yloop"() -> (w268:dbl)
                    n256 = Decrement(x=w268) -> (x-1=w269:dbl)
                    n257 = local read "Y序"() -> (w255:i32)
                    n258 = Replace Array Subset(array=w257, new element=w256, index (col)=w255) -> (w258:dbl[][])  [unwired: 1 in]
                    n259 = property on="强度图" class="IntGraph (严格)"("Value"=w258) -> ()  [unwired: 2 in, 2 out]
                    n260 = Equal?(x=w255, y=w269) -> (x = y?=w275:bool)
                    n261 = Increment(x=w255) -> ()  [unwired: 1 out]
                    n262 = flat-sequence {
                      tunnel: w251 -> [w281]
                      tunnel: [w281] -> w250
                      frame #0 {
                        n263 = local read "毫秒计时值"() -> (w276:u32)
                        n264 = Tick Count (ms)() -> (millisecond timer value=w280:u32)
                        n265 = Subtract(x=w280, y=w276) -> (x-y=w277:u32)
                        n266 = Multiply(x=w277, y=0.001) -> (x*y=→"已用时（s）":dbl)
                      }
                    }
                    n267 = property on="细分设置" class="DigNum (严格)"() -> ("Value"=w261:dbl)  [unwired: 2 in, 2 out]
                    n268 = property on="等待时间" class="DigNum (严格)"() -> ("Value"=w262:u32)  [unwired: 2 in, 2 out]
                    n269 = case shown="假" w275 {
                      tunnel: w250 -> [w359 w391]
                      tunnel: [w357 w392] -> w273
                      tunnel: w262 -> [w355 w389]
                      tunnel: w261 -> [w354 w388]
                      frame False {
                        n270 = flat-sequence {
                          tunnel: w359 -> [w363]
                          tunnel: [w363] -> w358
                          tunnel: [w361] -> w356
                          tunnel: w355 -> [w362]
                          tunnel: w354 -> [w361]
                          frame #0 {
                            n271 = call "X,Y,Z轴坐标查询.vi"("细分设置"=w361, "查询坐标轴"="Y", "串口通信端口"=w363) -> ("坐标(mm)"=w364:dbl)
                            n272 = property on="Y:" class="DigNum (严格)"() -> ("Value"=w360:dbl)  [unwired: 2 in, 2 out]
                            n273 = Add(x=w364, y=w360) -> (x+y=w366:dbl)
                            "x+y 2" <- w366
                            n274 = Multiply(x=w366, y=200.0) -> (x*y=w370:dbl)
                            n275 = Multiply(x=w370, y=8.0 ("细分设置")) -> (x*y=w375:dbl)
                            n276 = Number To Fractional String(number=w375, precision (6)=i16 0 ("精度(6)")) -> (F-format string=w373:string)  [unwired: 2 out]
                            n277 = Concatenate Strings("Y=" ("字符串"), w373, "/" ("字符串")) -> (w368:string)
                            n278 = call "步进电机命令输入与输出.vi"("输入字符串"=w368, "串口通信端口"=w363) -> ()  [unwired: 1 out]
                            n279 = Wait (ms)(milliseconds to wait=w362) -> ()  [unwired: 1 out]
                          }
                        }
                        n280 = while {
                          shift-right: [w377] -> w357
                          shift-left: w358 -> [w377]
                          shift-right: [w376] -> _
                          shift-left: w356 -> [w376]
                          stop <- w383 stop-if-true
                          n281 = call "X,Y,Z轴坐标查询.vi"("细分设置"=w376, "查询坐标轴"="Y", "串口通信端口"=w377) -> ("坐标(mm)"=w381:dbl)
                          n282 = local read "x+y 2"() -> (w384:dbl)
                          n283 = property on="电机急停" class="Bool (严格)"() -> ("Value"=w380:bool)  [unwired: 2 in, 2 out]
                          n284 = property on="Y(mm)" class="DigNum (严格)"("Value"=w381) -> ()  [unwired: 2 in, 2 out]
                          n285 = case shown="真" w380 {
                            tunnel: w377 -> [_ w386]
                            frame False {
                            }
                            frame True {
                              n286 = call "步进电机命令输入与输出.vi"("输入字符串"="S0/", "串口通信端口"=w386) -> ()  [unwired: 1 out]
                            }
                          }
                          n287 = Subtract(x=w384, y=w381) -> (x-y=w379:dbl)
                          n288 = Absolute Value(x=w379) -> (abs(x)=w378:dbl)
                          n289 = local read "精度"() -> (w382:dbl)
                          n290 = Less?(x=w378, y=w382) -> (x < y?=w383:bool)
                        }
                      }
                      frame True {
                        n291 = flat-sequence {
                          tunnel: [w396] -> _
                          tunnel: [w396] -> w393
                          tunnel: w391 -> [w396]
                          tunnel: [w394] -> w390
                          tunnel: w389 -> [w395]
                          tunnel: w388 -> [w394]
                          frame #0 {
                            n292 = Multiply(x=0.0, y=200.0) -> (x*y=w400:dbl)
                            n293 = Multiply(x=w400, y=w394) -> (x*y=w405:dbl)
                            n294 = Number To Fractional String(number=w405, precision (6)=i16 0 ("精度(6)")) -> (F-format string=w403:string)  [unwired: 2 out]
                            n295 = Concatenate Strings("Y=" ("字符串"), w403, "/" ("字符串")) -> (w398:string)
                            n296 = call "步进电机命令输入与输出.vi"("输入字符串"=w398, "串口通信端口"=w396) -> ()  [unwired: 1 out]
                            n297 = Wait (ms)(milliseconds to wait=w395) -> ()  [unwired: 1 out]
                          }
                        }
                        n298 = while {
                          shift-right: [w407] -> w392
                          shift-left: w393 -> [w407]
                          shift-right: [w406] -> _
                          shift-left: w390 -> [w406]
                          stop <- w413 stop-if-true
                          n299 = property on="电机急停" class="Bool (严格)"() -> ("Value"=w414:bool)  [unwired: 2 in, 2 out]
                          n300 = call "X,Y,Z轴坐标查询.vi"("细分设置"=w406, "查询坐标轴"="Y", "串口通信端口"=w407) -> ("坐标(mm)"=w415:dbl)
                          n301 = case shown="真" w414 {
                            tunnel: w407 -> [_ w418]
                            frame False {
                            }
                            frame True {
                              n302 = call "步进电机命令输入与输出.vi"("输入字符串"="S0/", "串口通信端口"=w418) -> ()  [unwired: 1 out]
                            }
                          }
                          n303 = Multiply(x=w415, y=1.0 ("x")) -> (x*y=w411:dbl)
                          n304 = Subtract(x=w411, y=0.0 ("x")) -> (x-y=w409:dbl)
                          n305 = local read "精度"() -> (w412:dbl)
                          n306 = Absolute Value(x=w409) -> (abs(x)=w408:dbl)
                          n307 = property on="Y(mm)" class="DigNum (严格)"("Value"=w411) -> ()  [unwired: 2 in, 2 out]
                          n308 = Less?(x=w408, y=w412) -> (x < y?=w413:bool)
                        }
                      }
                    }
                    "Y序" <- w274
                  }
                  n309 = property on="已用时（s）" class="DigNum (严格)"("Visible"=TRUE ("可见")) -> ()  [unwired: 2 in, 2 out]
                  n310 = flat-sequence {
                    tunnel: [w199] -> w182
                    tunnel: ["文件保存"] -> w180
                    tunnel: w180 -> [w204]
                    tunnel: [w203] -> w179
                    frame #0 {
                      n311 = Build Path(base path="文件保存", name or relative path="频域谱" ("名称或相对路径")) -> (appended path=w202:path)
                      n312 = Create Folder(path (use dialog)=w202) -> (created path=w199:path)  [unwired: 2 in, 2 out]
                    }
                    frame #1 {
                      n313 = Build Path(base path=w204, name or relative path="时域谱" ("名称或相对路径")) -> (appended path=w205:path)
                      n314 = Create Folder(path (use dialog)=w205) -> (created path=w203:path)  [unwired: 2 in, 2 out]
                    }
                  }
                  n315 = flat-sequence {
                    tunnel: w194 -> [w209]
                    tunnel: [w207] -> _
                    tunnel: [w207] -> w176
                    tunnel: [w209] -> w175
                    tunnel: w174 -> [w207]
                    tunnel: [w210] -> w193
                    tunnel: w176 -> [w210]
                    tunnel: w175 -> [w213]
                    frame #0 {
                      n316 = property on="水平进度条" class="Slide (严格)"("Value"=u8 100 ("水平进度条")) -> ()  [unwired: 2 in, 2 out]
                    }
                    frame #1 {
                      n317 = local read "毫秒计时值"() -> (w212:u32)
                      n318 = Tick Count (ms)() -> (millisecond timer value=w217:u32)
                      n319 = Transpose 2D Array(2D array=w213) -> (transposed array=w214:dbl[][])
                      n320 = Subtract(x=w217, y=w212) -> (x-y=w215:u32)
                      n321 = property on="强度图" class="IntGraph (严格)"("Value"=w214) -> ()  [unwired: 2 in, 2 out]
                      n322 = Multiply(x=w215, y=0.001) -> (x*y=w211:dbl)
                      n323 = property on="已用时（s）" class="DigNum (严格)"("Value"=w211) -> ()  [unwired: 2 in, 2 out]
                      "数组" <- w213
                    }
                  }
                }
                event "逐行扫描": Value Change {
                  n324 = event-data() -> ()  [unwired: 1 in, 6 out]
                  n325 = flat-sequence {
                    tunnel: [w573] -> w512
                    tunnel: [w572] -> w509
                    tunnel: w512 -> [w577]
                    tunnel: [w576] -> w511
                    frame #0 {
                      n326 = local read "文件保存"() -> (w573:path)
                      n327 = Build Path(base path=w573, name or relative path="频域谱" ("名称或相对路径")) -> (appended path=w575:path)
                      n328 = Create Folder(path (use dialog)=w575) -> (created path=w572:path)  [unwired: 2 in, 2 out]
                    }
                    frame #1 {
                      n329 = Build Path(base path=w577, name or relative path="时域谱" ("名称或相对路径")) -> (appended path=w578:path)
                      n330 = Create Folder(path (use dialog)=w578) -> (created path=w576:path)  [unwired: 2 in, 2 out]
                    }
                  }
                  n331 = flat-sequence {
                    tunnel: w507 -> [w530]
                    tunnel: [w530] -> w506
                    frame #0 {
                      # "如果强度图那里出了错，就把这里的行列互换"
                      n332 = property on="Y起点" class="DigNum (严格)"() -> ("Value"=w533:dbl)  [unwired: 2 in, 2 out]
                      n333 = property on="细分设置" class="DigNum (严格)"() -> ("Value"=w531:dbl)  [unwired: 2 in, 2 out]
                      n334 = local read "Xloop"() -> (w537:dbl)
                      n335 = local read "Yloop"() -> (w536:dbl)
                      n336 = Multiply(x=w533, y=200.0) -> (x*y=w541:dbl)
                      n337 = Tick Count (ms)() -> (millisecond timer value=w534:u32)
                      n338 = Multiply(x=w541, y=w531) -> (x*y=w546:dbl)
                      n339 = Initialize Array(0.0 ("元素"), w537, w536) -> (w532:dbl[][])
                      n340 = Number To Fractional String(number=w546, precision (6)=i16 0 ("精度(6)")) -> (F-format string=w544:string)  [unwired: 2 out]
                      n341 = property on="毫秒计时值" class="DigNum (严格)"("Value"=w534) -> ()  [unwired: 2 in, 2 out]
                      n342 = property on="强度图" class="IntGraph (严格)"("Value"=w532) -> ()  [unwired: 2 in, 2 out]
                      n343 = Concatenate Strings("Y=" ("字符串"), w544, "/" ("字符串")) -> (w539:string)
                      n344 = call "步进电机命令输入与输出.vi"("输入字符串"=w539, "串口通信端口"=w530) -> ()  [unwired: 1 out]
                      n345 = property on="等待时间" class="DigNum (严格)"() -> ("Value"=w535:u32)  [unwired: 2 in, 2 out]
                      n346 = property on="已用时（s）" class="DigNum (严格)"("Value"=0.0 ("已用时（s）")) -> ()  [unwired: 2 in, 2 out]
                      n347 = Wait (ms)(milliseconds to wait=w535) -> ()  [unwired: 1 out]
                    }
                  }
                  n348 = property on="水平进度条" class="Slide (严格)"("Visible"=TRUE ("可见")) -> ()  [unwired: 2 in, 2 out]
                  n349 = flat-sequence {
                    tunnel: [w525] -> w505
                    frame #0 {
                      n350 = property on="X终点" class="DigNum (严格)"() -> ("Value"=w514:dbl)  [unwired: 2 in, 2 out]
                      n351 = property on="X起点" class="DigNum (严格)"() -> ("Value"=w513:dbl)  [unwired: 2 in, 2 out]
                      n352 = Subtract(x=w514, y=w513) -> (x-y=w518:dbl)
                      n353 = local read "X:"() -> (w517:dbl)
                      n354 = property on="X扫描范围" class="DigNum (严格)"("Value"=w518) -> ()  [unwired: 2 in, 2 out]
                      n355 = Divide(x=w518, y=w517) -> (x/y=w516:dbl)
                      n356 = Increment(x=w516) -> (x+1=w515:dbl)
                      n357 = property on="Xloop" class="DigNum (严格)"("Value"=w515) -> ()  [unwired: 2 in, 2 out]
                    }
                    frame #1 {
                      n358 = property on="Y终点" class="DigNum (严格)"() -> ("Value"=w520:dbl)  [unwired: 2 in, 2 out]
                      n359 = property on="Y起点" class="DigNum (严格)"() -> ("Value"=w519:dbl)  [unwired: 2 in, 2 out]
                      n360 = Subtract(x=w520, y=w519) -> (x-y=w523:dbl)
                      n361 = local read "Y:"() -> (w522:dbl)
                      n362 = property on="Y扫描范围" class="DigNum (严格)"("Value"=w523) -> ()  [unwired: 2 in, 2 out]
                      n363 = Divide(x=w523, y=w522) -> (x/y=w524:dbl)
                      n364 = Increment(x=w524) -> (x+1=w521:dbl)
                      n365 = property on="Yloop" class="DigNum (严格)"("Value"=w521) -> ()  [unwired: 2 in, 2 out]
                    }
                    frame #2 {
                      n366 = property on="Xloop" class="DigNum (严格)"() -> ("Value"=w528:dbl)  [unwired: 2 in, 2 out]
                      n367 = property on="Yloop" class="DigNum (严格)"() -> ("Value"=w525:dbl)  [unwired: 2 in, 2 out]
                      n368 = Initialize Array(0.0 ("元素"), w528, w525) -> (w527:dbl[][])
                      n369 = property on="强度图" class="IntGraph (严格)"("Value"=w527) -> ()  [unwired: 2 in, 2 out]
                    }
                  }
                  n370 = while {
                    shift-right: [w548] -> w508
                    shift-left: w506 -> [w548]
                    stop <- w553 stop-if-true
                    n371 = call "X,Y,Z轴坐标查询.vi"("细分设置"=8.0, "查询坐标轴"="Y", "串口通信端口"=w548) -> ("坐标(mm)"=w555:dbl)
                    n372 = property on="Y起点" class="DigNum (严格)"() -> ("Value"=w547:dbl)  [unwired: 2 in, 2 out]
                    n373 = property on="电机急停" class="Bool (严格)"() -> ("Value"=w554:bool)  [unwired: 2 in, 2 out]
                    n374 = Multiply(x=w555, y=1.0 ("x")) -> (x*y=w551:dbl)
                    n375 = Subtract(x=w547, y=w551) -> (x-y=w550:dbl)
                    n376 = case shown="真" w554 {
                      tunnel: w548 -> [_ w559]
                      frame False {
                      }
                      frame True {
                        n377 = call "步进电机命令输入与输出.vi"("输入字符串"="S0/", "串口通信端口"=w559) -> ()  [unwired: 1 out]
                      }
                    }
                    n378 = Absolute Value(x=w550) -> (abs(x)=w549:dbl)
                    n379 = local read "精度"() -> (w552:dbl)
                    n380 = property on="Y(mm)" class="DigNum (严格)"("Value"=w551) -> ()  [unwired: 2 in, 2 out]
                    n381 = Less?(x=w549, y=w552) -> (x < y?=w553:bool)
                  }
                  n382 = for {
                    N: w505 -> [_]
                    shift-right: [w597] -> _
                    shift-left: w509 -> [w597]
                    shift-right: [w596] -> _
                    shift-left: w511 -> [w596]
                    tunnel: [w595] -> w504 mode=indexing
                    shift-right: [w585] -> w503
                    shift-left: w508 -> [w587]
                    i -> [w580]
                    # "实时成像出问题调这里"
                    n383 = property on="Y序" class="DigNum (严格)"("Value"=w580) -> ()  [unwired: 2 in, 2 out]
                    n384 = local read "Yloop"() -> (w582:dbl)
                    n385 = Multiply(x=w582, y=0.01) -> (x*y=w581:dbl)
                    n386 = Divide(x=w580, y=w581) -> (x/y=w583:dbl)
                    n387 = property on="水平进度条" class="Slide (严格)"("Value"=w583) -> ()  [unwired: 2 in, 2 out]
                    n388 = flat-sequence {
                      tunnel: [w640] -> w600
                      tunnel: [w638] -> w599
                      tunnel: [w641] -> w595
                      tunnel: [w639] -> w598
                      tunnel: w587 -> [w637]
                      tunnel: [w671] -> w591
                      tunnel: w596 -> [w655]
                      tunnel: w597 -> [w654]
                      tunnel: w600 -> [w667]
                      tunnel: w599 -> [w671]
                      tunnel: w598 -> [w659]
                      frame #0 {
                        n389 = local read "精度"() -> (w649:dbl)
                        n390 = property on="细分设置" class="DigNum (严格)"() -> ("Value"=w648:dbl)  [unwired: 2 in, 2 out]
                        n391 = property on="X终点" class="DigNum (严格)"() -> ("Value"=w652:dbl)  [unwired: 2 in, 2 out]
                        n392 = property on="X起点" class="DigNum (严格)"() -> ("Value"=w636:dbl)  [unwired: 2 in, 2 out]
                        n393 = local read "pulDDR2Length"() -> (w644:u32)
                        n394 = local read "M_Length"() -> (w646:i32)
                        n395 = property on="hDevice" class="DigNum (严格)"() -> ("Value"=w645:i32)  [unwired: 2 in, 2 out]
                        n396 = property on="N_Length" class="DigNum (严格)"() -> ("Value"=w647:i32)  [unwired: 2 in, 2 out]
                        n397 = property on="等待时间" class="DigNum (严格)"() -> ("Value"=w650:u32)  [unwired: 2 in, 2 out]
                        n398 = property on="电机急停" class="Bool (严格)"() -> ("Value"=w651:bool)  [unwired: 2 in, 2 out]
                        n399 = call "X轴连续扫描（1.0）.vi"("VISA I"=w637, "X0"=w636, "X"=w652, "精度"=w649, "细分设置"=w648, "等待时间(ms)"=w650, "pulDDR2Length"=w644, "电机急停"=w651, "hDevice"=w645, "M-length"=w646, "N-length"=w647) -> ("VISA O"=w638:refnum<visa-resource-name>, "hDevice out"=w643:i32, "X"=w642:dbl, "强度图行"=w641:dbl[], "时域谱页"=w640:dbl[][], "幅频谱页"=w639:dbl[][])  [unwired: 3 in]
                        n400 = property on="hDevice 2" class="DigNum (严格)"("Value"=w643) -> ()  [unwired: 2 in, 2 out]
                        n401 = property on="X（mm）" class="DigNum (严格)"("Value"=w642) -> ()  [unwired: 2 in, 2 out]
                      }
                      frame #1 {
                        n402 = property on="Y序" class="DigNum (严格)"() -> ("Value"=w653:i32)  [unwired: 2 in, 2 out]
                        n403 = Increment(x=w653) -> (x+1=w656:i32)
                        n404 = Number To Decimal String(number=w656) -> (decimal integer string=w665:string)  [unwired: 1 in]
                        n405 = Number To Decimal String(number=w656) -> (decimal integer string=w664:string)  [unwired: 1 in]
                        n406 = Concatenate Strings("T" ("字符串"), w665, ".txt" ("字符串")) -> (w668:string)
                        n407 = Concatenate Strings("F" ("字符串"), w664, ".txt" ("字符串")) -> (w662:string)
                        n408 = Build Path(base path=w655, name or relative path=w668) -> (appended path=w670:path)
                        n409 = call-poly <vilib>:"Write Delimited Spreadsheet.vi"("file path (dialog if empty)"=w670, "2D data"=w667, "transpose? (no:F)"=FALSE) -> ()  [unwired: 11 in, 2 out]
                        n410 = Build Path(base path=w654, name or relative path=w662) -> (appended path=w660:path)
                        n411 = call-poly <vilib>:"Write Delimited Spreadsheet.vi"("file path (dialog if empty)"=w660, "2D data"=w659, "transpose? (no:F)"=FALSE) -> ()  [unwired: 11 in, 2 out]
                      }
                    }
                    n412 = flat-sequence {
                      tunnel: w591 -> [w613]
                      tunnel: [w613] -> w592
                      tunnel: [w612] -> w593
                      frame #0 {
                        n413 = property on="细分设置" class="DigNum (严格)"() -> ("Value"=w612:dbl)  [unwired: 2 in, 2 out]
                        n414 = Multiply(x=0.0, y=50.0) -> (x*y=w616:dbl)
                        n415 = Multiply(x=w616, y=w612) -> (x*y=w621:dbl)
                        n416 = local read "等待时间"() -> (w611:u32)
                        n417 = Number To Fractional String(number=w621, precision (6)=i16 0 ("精度(6)")) -> (F-format string=w619:string)  [unwired: 2 out]
                        n418 = Concatenate Strings("X=" ("字符串"), w619, "/" ("字符串")) -> (w614:string)
                        n419 = Wait (ms)(milliseconds to wait=w611) -> ()  [unwired: 1 out]
                        n420 = call "步进电机命令输入与输出.vi"("输入字符串"=w614, "串口通信端口"=w613) -> ()  [unwired: 1 out]
                      }
                    }
                    n421 = while {
                      shift-right: [w625] -> w590
                      shift-left: w592 -> [w625]
                      shift-right: [w623] -> _
                      shift-left: w593 -> [w623]
                      stop <- w629 stop-if-true
                      n422 = property on="电机急停" class="Bool (严格)"() -> ("Value"=w630:bool)  [unwired: 2 in, 2 out]
                      n423 = case shown="真" w630 {
                        tunnel: w625 -> [_ w634]
                        frame False {
                        }
                        frame True {
                          n424 = call "步进电机命令输入与输出.vi"("输入字符串"="S0/", "串口通信端口"=w634) -> ()  [unwired: 1 out]
                        }
                      }
                      n425 = call "X,Y,Z轴坐标查询.vi"("细分设置"=w623, "查询坐标轴"="X", "串口通信端口"=w625) -> ("坐标(mm)"=w631:dbl)
                      n426 = Multiply(x=w631, y=4.0 ("x")) -> (x*y=w627:dbl)
                      n427 = Subtract(x=0.0, y=w627) -> (x-y=w626:dbl)
                      n428 = local read "精度"() -> (w628:dbl)
                      n429 = Absolute Value(x=w626) -> (abs(x)=w624:dbl)
                      n430 = property on="X（mm）" class="DigNum (严格)"("Value"=w627) -> ()  [unwired: 2 in, 2 out]
                      n431 = Less?(x=w624, y=w628) -> (x < y?=w629:bool)
                    }
                    n432 = property on="强度图" class="IntGraph (严格)"() -> ("Value"=w603:dbl[][])  [unwired: 2 in, 2 out]
                    n433 = property on="Yloop" class="DigNum (严格)"() -> ("Value"=w588:dbl)  [unwired: 2 in, 2 out]
                    n434 = property on="Y序" class="DigNum (严格)"() -> ("Value"=w594:i32)  [unwired: 2 in, 2 out]
                    n435 = Replace Array Subset(array=w603, new element=w595, index (col)=w594) -> (w602:dbl[][])  [unwired: 1 in]
                    n436 = property on="强度图" class="IntGraph (严格)"("Value"=w602) -> ()  [unwired: 2 in, 2 out]
                    n437 = Decrement(x=w588) -> (x-1=w589:dbl)
                    n438 = Equal?(x=w594, y=w589) -> (x = y?=w601:bool)
                    n439 = case shown="假" w601 {
                      tunnel: w590 -> [w675 w705]
                      tunnel: [w673 w706] -> w586
                      frame False {
                        n440 = flat-sequence {
                          tunnel: w675 -> [w679]
                          tunnel: [w679] -> w674
                          tunnel: [w676] -> w672
                          frame #0 {
                            n441 = property on="细分设置" class="DigNum (严格)"() -> ("Value"=w676:dbl)  [unwired: 2 in, 2 out]
                            n442 = call "X,Y,Z轴坐标查询.vi"("细分设置"=w676, "查询坐标轴"="Y", "串口通信端口"=w679) -> ("坐标(mm)"=w680:dbl)
                            n443 = property on="Y:" class="DigNum (严格)"() -> ("Value"=w678:dbl)  [unwired: 2 in, 2 out]
                            n444 = Add(x=w680, y=w678) -> (x+y=w682:dbl)
                            "x+y 3" <- w682
                            n445 = Multiply(x=w682, y=200.0) -> (x*y=w686:dbl)
                            n446 = Multiply(x=w686, y=8.0 ("细分设置")) -> (x*y=w691:dbl)
                            n447 = Number To Fractional String(number=w691, precision (6)=i16 0 ("精度(6)")) -> (F-format string=w689:string)  [unwired: 2 out]
                            n448 = Concatenate Strings("Y=" ("字符串"), w689, "/" ("字符串")) -> (w684:string)
                            n449 = call "步进电机命令输入与输出.vi"("输入字符串"=w684, "串口通信端口"=w679) -> ()  [unwired: 1 out]
                            n450 = property on="等待时间" class="DigNum (严格)"() -> ("Value"=w677:u32)  [unwired: 2 in, 2 out]
                            n451 = Wait (ms)(milliseconds to wait=w677) -> ()  [unwired: 1 out]
                          }
                        }
                        n452 = while {
                          shift-right: [w694] -> w673
                          shift-left: w674 -> [w694]
                          shift-right: [w693] -> _
                          shift-left: w672 -> [w693]
                          stop <- w700 stop-if-true
                          n453 = call "X,Y,Z轴坐标查询.vi"("细分设置"=w693, "查询坐标轴"="Y", "串口通信端口"=w694) -> ("坐标(mm)"=w698:dbl)
                          n454 = property on="x+y 3" class="DigNum (严格)"() -> ("Value"=w692:dbl)  [unwired: 2 in, 2 out]
                          n455 = property on="电机急停" class="Bool (严格)"() -> ("Value"=w697:bool)  [unwired: 2 in, 2 out]
                          n456 = property on="Y(mm)" class="DigNum (严格)"("Value"=w698) -> ()  [unwired: 2 in, 2 out]
                          n457 = case shown="真" w697 {
                            tunnel: w694 -> [_ w702]
                            frame False {
                            }
                            frame True {
                              n458 = call "步进电机命令输入与输出.vi"("输入字符串"="S0/", "串口通信端口"=w702) -> ()  [unwired: 1 out]
                            }
                          }
                          n459 = Subtract(x=w692, y=w698) -> (x-y=w696:dbl)
                          n460 = Absolute Value(x=w696) -> (abs(x)=w695:dbl)
                          n461 = local read "精度"() -> (w699:dbl)
                          n462 = Less?(x=w695, y=w699) -> (x < y?=w700:bool)
                        }
                      }
                      frame True {
                        n463 = flat-sequence {
                          tunnel: [w710] -> _
                          tunnel: [w710] -> w707
                          tunnel: w705 -> [w710]
                          tunnel: [w708] -> w704
                          frame #0 {
                            n464 = property on="细分设置" class="DigNum (严格)"() -> ("Value"=w708:dbl)  [unwired: 2 in, 2 out]
                            n465 = Multiply(x=0.0, y=200.0) -> (x*y=w714:dbl)
                            n466 = Multiply(x=w714, y=w708) -> (x*y=w719:dbl)
                            n467 = Number To Fractional String(number=w719, precision (6)=i16 0 ("精度(6)")) -> (F-format string=w717:string)  [unwired: 2 out]
                            n468 = Concatenate Strings("Y=" ("字符串"), w717, "/" ("字符串")) -> (w712:string)
                            n469 = call "步进电机命令输入与输出.vi"("输入字符串"=w712, "串口通信端口"=w710) -> ()  [unwired: 1 out]
                            n470 = property on="等待时间" class="DigNum (严格)"() -> ("Value"=w709:u32)  [unwired: 2 in, 2 out]
                            n471 = Wait (ms)(milliseconds to wait=w709) -> ()  [unwired: 1 out]
                          }
                        }
                        n472 = while {
                          shift-right: [w721] -> w706
                          shift-left: w707 -> [w721]
                          shift-right: [w720] -> _
                          shift-left: w704 -> [w720]
                          stop <- w727 stop-if-true
                          n473 = property on="电机急停" class="Bool (严格)"() -> ("Value"=w728:bool)  [unwired: 2 in, 2 out]
                          n474 = call "X,Y,Z轴坐标查询.vi"("细分设置"=w720, "查询坐标轴"="Y", "串口通信端口"=w721) -> ("坐标(mm)"=w729:dbl)
                          n475 = case shown="真" w728 {
                            tunnel: w721 -> [_ w732]
                            frame False {
                            }
                            frame True {
                              n476 = call "步进电机命令输入与输出.vi"("输入字符串"="S0/", "串口通信端口"=w732) -> ()  [unwired: 1 out]
                            }
                          }
                          n477 = Multiply(x=w729, y=1.0 ("x")) -> (x*y=w725:dbl)
                          n478 = Subtract(x=w725, y=0.0 ("x")) -> (x-y=w723:dbl)
                          n479 = local read "精度"() -> (w726:dbl)
                          n480 = Absolute Value(x=w723) -> (abs(x)=w722:dbl)
                          n481 = property on="Y(mm)" class="DigNum (严格)"("Value"=w725) -> ()  [unwired: 2 in, 2 out]
                          n482 = Less?(x=w722, y=w726) -> (x < y?=w727:bool)
                        }
                      }
                    }
                    n483 = flat-sequence {
                      tunnel: w586 -> [w604]
                      tunnel: [w604] -> w585
                      frame #0 {
                        n484 = local read "毫秒计时值"() -> (w605:u32)
                        n485 = Tick Count (ms)() -> (millisecond timer value=w608:u32)
                        n486 = Subtract(x=w608, y=w605) -> (x-y=w606:u32)
                        n487 = Multiply(x=w606, y=0.001) -> (x*y=w609:dbl)
                        n488 = property on="已用时（s）" class="DigNum (严格)"("Value"=w609) -> ()  [unwired: 2 in, 2 out]
                      }
                    }
                  }
                  n489 = property on="已用时（s）" class="DigNum (严格)"("Visible"=TRUE ("可见")) -> ()  [unwired: 2 in, 2 out]
                  n490 = flat-sequence {
                    tunnel: w504 -> [w562]
                    tunnel: w503 -> [w563]
                    tunnel: [w563] -> w500
                    tunnel: [w562] -> w499
                    tunnel: [w565] -> w510
                    tunnel: w500 -> [w565]
                    tunnel: w499 -> [w566]
                    frame #0 {
                      n491 = property on="水平进度条" class="Slide (严格)"("Value"=u8 100 ("水平进度条")) -> ()  [unwired: 2 in, 2 out]
                    }
                    frame #1 {
                      n492 = local read "毫秒计时值"() -> (w570:u32)
                      n493 = property on="数组" class="Arr (严格)"("Value"=w566) -> ()  [unwired: 2 in, 2 out]
                      n494 = Transpose 2D Array(2D array=w566) -> (transposed array=w567:dbl[][])
                      n495 = Tick Count (ms)() -> (millisecond timer value=w571:u32)
                      n496 = property on="强度图" class="IntGraph (严格)"("Value"=w567) -> ()  [unwired: 2 in, 2 out]
                      n497 = Subtract(x=w571, y=w570) -> (x-y=w568:u32)
                      n498 = Multiply(x=w568, y=0.001) -> (x*y=w564:dbl)
                      n499 = property on="已用时（s）" class="DigNum (严格)"("Value"=w564) -> ()  [unwired: 2 in, 2 out]
                    }
                  }
                }
                event "分层图查看": Value Change {
                  n500 = event-data() -> ()  [unwired: 1 in, 6 out]
                  n501 = call "分层图显示1.1.vi"("IN"=w735) -> ("OUT"=w734:string)  [unwired: 10 in]
                }
              }
            }
          }
        }
        n502 = flat-sequence {
          tunnel: w22 -> [w60]
          frame #0 {
            n503 = dll-call lib="PTH2]abs CUsersH301Desktopart闭环扫描程序采集卡控制INFamd64\nPCI8502_32" fn="PCI8502_ReleaseDeviceAD" label="ReleaseDeviceAD"("hDevice"="hDevice 2") -> ("hDevice"=w62:i32)  [unwired: 4 in, 2 out]
            n504 = VISA Close(VISA resource name=w60) -> (error out=→"错误输出":errorcluster)  [unwired: 1 in]
            n505 = dll-call lib="PTH2]abs CUsersH301Desktopart闭环扫描程序采集卡控制INFamd64\nPCI8502_32" fn="PCI8502_ReleaseDevice" label="ReleaseDevice"("hDevice"=w62) -> ()  [unwired: 5 in, 2 out]
          }
          frame #1 {
            n506 = Request Deallocation(TRUE ("标志")) -> ()
          }
        }
        "M_Length" <- w26
      }
    }
  }
  n507 = property on="高级设置" class="Bool"("Visible"=FALSE ("可见")) -> ()  [unwired: 2 in, 2 out]
  n508 = property on="定位模式" class="Bool"("Visible"=FALSE ("可见")) -> ()  [unwired: 2 in, 2 out]
  n509 = property on="已用时（s）" class="DigNum (严格)"("Visible"=FALSE ("可见")) -> ()  [unwired: 2 in, 2 out]
